vi "File.List Files and SubFolders.vi"(8 "error in":errorcluster, 10 "Pattern":string, 11 "Folder":path) -> (0 "error out":errorcluster, 2 "Folders":path[](array[path]), 3 "Files":path[](array[path]))   [LabVIEW 2024, in "EQMF.lvlib" / "File Utils.lvlib"]
uses:
  File Utils.lvlib
  <vilib>/Utility/error.llb/Trim Whitespace One-Sided.vi
  Status/Status Utils.lvlib
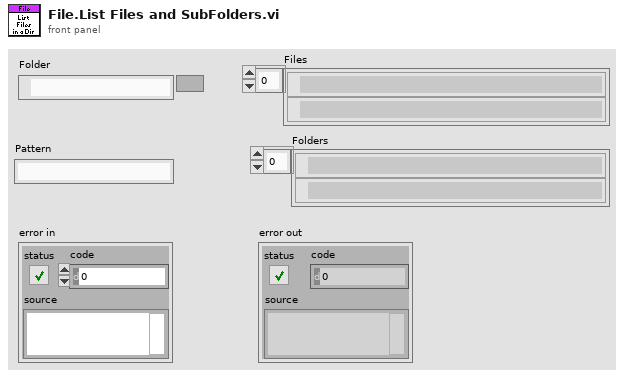
[diagram p1: front panel]
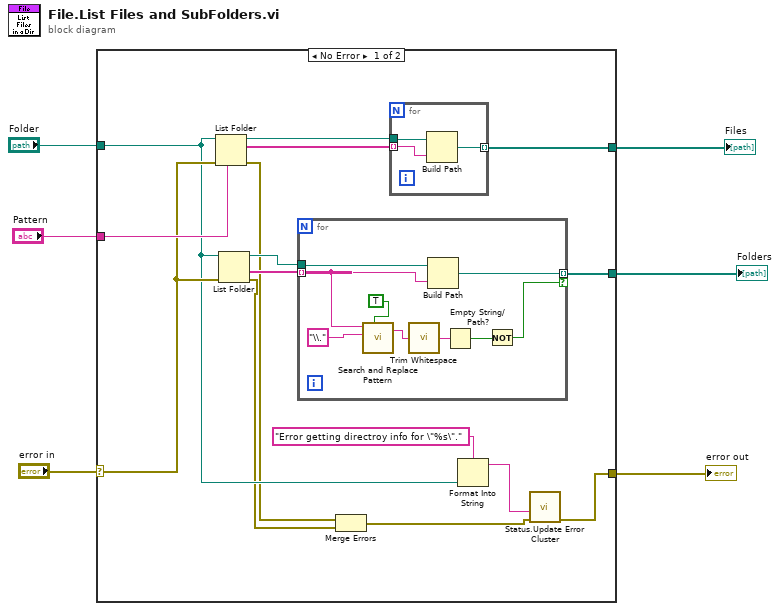
[diagram p0: block diagram]
diagram:
  n1 = case shown="No Error" "error in" {
    selector: "error in" -> [w16 w34]
    tunnel: [w19 _] -> w6
    tunnel: [w18 _] -> w5
    tunnel: [w7 w34] -> w4
    tunnel: "Pattern" -> [w17 _]
    tunnel: "Folder" -> [w11 _]
    frame No Error {
      n2 = List Folder(path=w11, pattern=w17, error in=w16) -> (path out=w20:path, filenames=w21:string[], error out=w9:errorcluster)  [unwired: 1 in, 1 out]
      n3 = List Folder(path=w11, error in=w16) -> (path out=w14:path, folder names=w15:string[], error out=w10:errorcluster)  [unwired: 2 in, 1 out]
      n4 = for {
        tunnel: w14 -> [w30]
        tunnel: w15 -> [w27] mode=indexing
        tunnel: [w29] -> w18 mode=indexing if=w24
        n5 = call <vilib>:"Search and Replace Pattern.vi"("string"=w27, "regular expression (\"\")"="\\." ("regular expression (\"\")"), "replace all? (F)"=TRUE) -> ("result string"=w22:string)  [unwired: 2 in, 1 out]
        n6 = call <vilib>:"Trim Whitespace.vi"("string"=w22) -> ("trimmed string"=w23:string)  [unwired: 1 in]
        n7 = Build Path(base path=w30, name or relative path=w27) -> (appended path=w29:path)
        n8 = Empty String/Path?(string/path=w23) -> (empty?=w28:bool)
        n9 = Not(x=w28) -> (.not. x?=w24:bool)
      }
      n10 = Merge Errors(w9, w10) -> (w8:errorcluster)
      n11 = for {
        tunnel: w20 -> [w33]
        tunnel: w21 -> [w32] mode=indexing
        tunnel: [w31] -> w19 mode=indexing
        n12 = Build Path(base path=w33, name or relative path=w32) -> (appended path=w31:path)
      }
      n13 = Format Into String(format string="Error getting directroy info for \"%s\".", w11) -> (resulting string=w12:string)  [unwired: 2 in, 1 out]
      n14 = call "Status.Update Error Cluster.vi"("Error In"=w8, "NewDesc"=w12) -> ("Error Out"=w7:errorcluster)  [unwired: 9 in]
    }
    frame Error {
    }
  }
  "Files" <- w6
  "Folders" <- w5
  "error out" <- w4
